vi "CMD_GETVECPOPUP.vi"(6 "Gantry in":refnum<class "Gantry.lvclass">, 8 "error in (no error)":errorcluster, 10 "Arguments":string[](array[string]), 11 "gScript Interpreter in":refnum<class "gScript Interpreter.lvclass">) -> (0 "error out":errorcluster, 3 "gScript Interpreter out":refnum<class "gScript Interpreter.lvclass">, 4 "Gantry out":refnum<class "Gantry.lvclass">)   [LabVIEW 2022 SP3, in "gScript Interpreter.lvclass"]
uses:
  gScript Interpreter.lvclass
  gScript Interpreter.lvclass/gScript Interpreter.ctl
  Shared Components/Vec3d Class/Vec3d.lvclass
  Shared Components/Gantry Class/Gantry.lvclass
panel:
  in  "Z":dbl caption="Input" format="%#g"
  in  "Y":dbl caption="Input" format="%#g"
  out "Message":string
  in  "X":dbl caption="Input" format="%#g"
  in  "OK":bool caption="OK1"
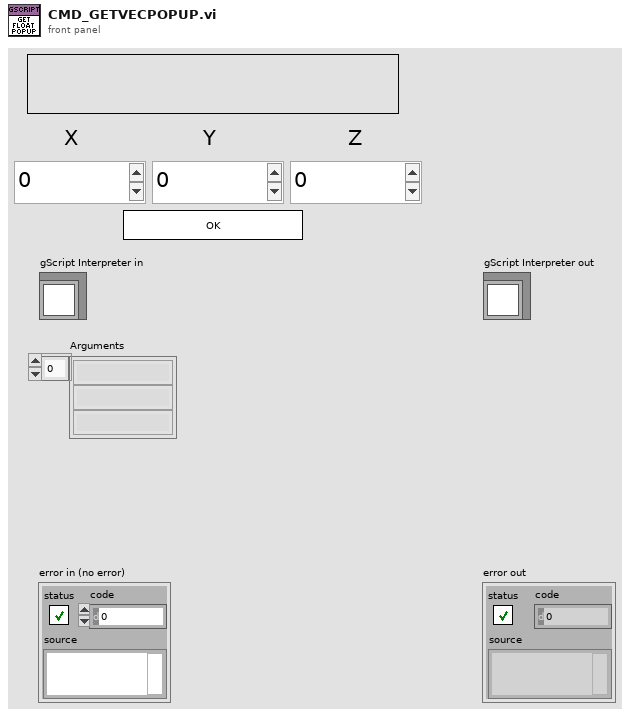
[diagram p1: front panel]
types:
  T1 = typedef "Memory Cell.ctl" = cluster{"type":T2, "x":dbl, "y":dbl, "z":dbl, "w":dbl}
  T2 = typedef "Memory Cell Type Enum.ctl" = enum16{"integer", "float", "vector", "rotation"}
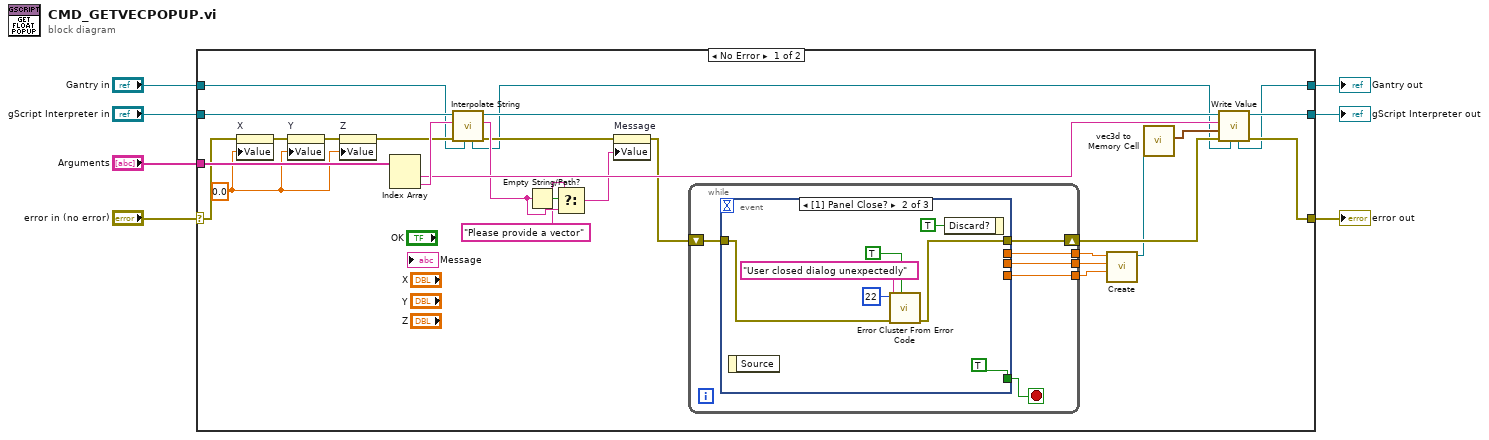
[diagram p0: block diagram]
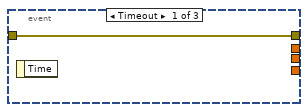
[diagram p2: hidden frame]
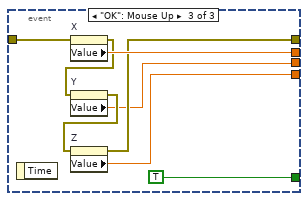
[diagram p3: hidden frame]
diagram:
  n1 = case shown="No Error" "error in (no error)" {
    selector: "error in (no error)" -> [w15 w59]
    tunnel: [w30 w59] -> w6
    tunnel: [w29 w58] -> w4
    tunnel: "gScript Interpreter in" -> [w33 w58]
    tunnel: "Arguments" -> [w34 _]
    tunnel: "Gantry in" -> [w10 w57]
    tunnel: [w8 w57] -> w1
    frame No Error {
      w11 = 0.0 ("X")
      n2 = property on="X" class="DigNum (strict)"(error in=w15, "Value"=w11) -> (error out=w14:errorcluster)  [unwired: 1 in, 1 out]
      n3 = property on="Y" class="DigNum (strict)"(error in=w14, "Value"=w11) -> (error out=w13:errorcluster)  [unwired: 1 in, 1 out]
      n4 = property on="Z" class="DigNum (strict)"(error in=w13, "Value"=w11) -> (error out=w12:errorcluster)  [unwired: 1 in, 1 out]
      n5 = Index Array(array=w34) -> (element #1=w31:string, element #2=w32:string)  [unwired: 2 in]
      n6 = call-dynamic "Interpolate String.vi"("Gantry in"=w10, "error in (no error)"=w12, "Input String"=w32, "gScript Interpreter in"=w33) -> ("error out"=w23:errorcluster, "Output String"=w27:string, "gScript Interpreter out"=w24:refnum<class "gScript Interpreter.lvclass">, "Gantry out"=w9:refnum<class "Gantry.lvclass">)  [unwired: 4 in]
      n7 = Empty String/Path?(string/path=w27) -> (empty?=w28:bool)
      n8 = Select(t="Please provide a vector", s=w28, f=w27) -> (s? t:f=w25:string)
      n9 = property on="Message" class="Str"(error in=w23, "Value"=w25) -> (error out=w22:errorcluster)  [unwired: 1 in, 1 out]
      n10 = while {
        shift-right: [w38] -> w21
        shift-left: w22 -> [w39]
        tunnel: [w37] -> w20
        tunnel: [w36] -> w19
        tunnel: [w35] -> w18
        stop <- w40 stop-if-true
        n11 = event shown="[1] Panel Close?" {
          selector: _ -> [_ _ _]
          dyn-events: _ -> [_ _ _]
          timeout: _ -> [_ _ _]
          tunnel: [_ TRUE TRUE] -> w40
          tunnel: w39 -> [w41 w45 w55]
          tunnel: [w41 w44 w51] -> w38
          tunnel: [_ _ w54] -> w37
          tunnel: [_ _ w50] -> w36
          tunnel: [_ _ w49] -> w35
          event Timeout {
            n12 = event-data() -> ()  [unwired: 1 in, 1 out]
          }
          event Panel Close? {
            n13 = event-data() -> ()  [unwired: 1 in, 1 out]
            n14 = call <vilib>:"Error Cluster From Error Code.vi"("show call chain? (False)"=TRUE, "error in (no error)"=w45, "error message (\"\")"="User closed dialog unexpectedly" ("error message (\"\")"), "error code (0)"=22) -> ("error out"=w44:errorcluster)  [unwired: 5 in]
            n15 = event-data("Discard?"=TRUE) -> ()  [unwired: 1 in, 1 out]
          }
          event "OK": Mouse Up {
            n16 = event-data() -> ()  [unwired: 1 in, 1 out]
            n17 = property on="X" class="DigNum (strict)"(error in=w55) -> (error out=w53:errorcluster, "Value"=w54:dbl)  [unwired: 1 in, 1 out]
            n18 = property on="Y" class="DigNum (strict)"(error in=w53) -> (error out=w52:errorcluster, "Value"=w50:dbl)  [unwired: 1 in, 1 out]
            n19 = property on="Z" class="DigNum (strict)"(error in=w52) -> (error out=w51:errorcluster, "Value"=w49:dbl)  [unwired: 1 in, 1 out]
          }
        }
      }
      n20 = call "Create.vi"("Z"=w18, "Y"=w19, "X"=w20) -> ("Vec3d Class out"=w17:refnum<class "Vec3d.lvclass">)  [unwired: 7 in, 1 out]
      n21 = call "vec3d to Memory Cell.vi"("Vec3d in"=w17) -> ("Memory Cell"=w16:T1)  [unwired: 10 in]
      n22 = call-dynamic "Write Value.vi"("Gantry in"=w9, "error in (no error)"=w21, "Value"=w16, "Address"=w31, "gScript Interpreter in"=w24) -> ("error out"=w30:errorcluster, "gScript Interpreter out"=w29:refnum<class "gScript Interpreter.lvclass">, "Gantry out"=w8:refnum<class "Gantry.lvclass">)  [unwired: 4 in]
    }
    frame Error {
    }
  }
  "error out" <- w6
  "gScript Interpreter out" <- w4
  "Gantry out" <- w1
